vi "ustaw kursor.vi"(6 "przesuniecie (10)":dbl=10.0 format="%#_13g", 8 "XScale.Maximum":dbl, 10 "XScale.Minimum":dbl, 11 "signal in":waveform(dbl)) -> (2 "dt x Index":dbl, 3 "Index":i32, 5 "dt":dbl)   [LabVIEW 2014]
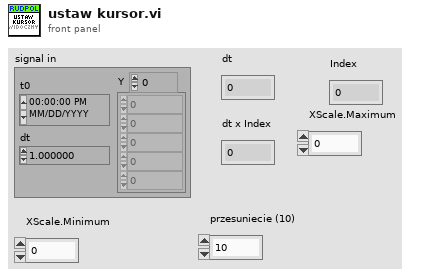
[diagram p1: front panel]
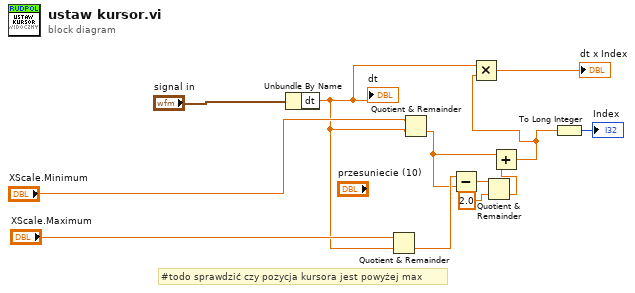
[diagram p0: block diagram]
diagram:
  # "#todo sprawdzić czy pozycja kursora jest powyżej max"
  n1 = Unbundle By Name("signal in") -> ("dt"=w7:dbl)
  "dt" <- w7
  n2 = Quotient & Remainder(x="XScale.Maximum", y=w7) -> (floor(x/y)=w6:dbl)  [unwired: 1 out]
  n3 = Quotient & Remainder(x="XScale.Minimum", y=w7) -> (floor(x/y)=w3:dbl)  [unwired: 1 out]
  n4 = Subtract(x=w6, y=w3) -> (x-y=w5:dbl)
  n5 = Quotient & Remainder(x=w5, y=2.0) -> (floor(x/y)=w2:dbl)  [unwired: 1 out]
  n6 = Add(x=w3, y=w2) -> (x+y=w1:dbl)
  n7 = Multiply(x=w7, y=w1) -> (x*y=→"dt x Index":dbl)
  n8 = To Long Integer(number=w1) -> (32bit integer=→"Index":i32)
